vi "Configure Power.vi"(0 "VISA resource name":refnum<visa-resource-name>, 1 "Power Reference (0 dBm)":dbl, 2 "Enable Power Reference (F:Disable)":bool, 5 "Power (-130 dBm)":dbl=-130.0, 7 "Power Offset (0 dB)":dbl, 9 "Attenuator Auto Mode (T:Enable)":bool=TRUE, 11 "error in (no error)":errorcluster, 12 "Enable Attenuator Bypass (F:Disable)":bool, 13 "Attenuation Level (115 dB)":dbl=115.0) -> (4 "VISA resource name out":refnum<visa-resource-name>, 15 "error out":errorcluster)   [LabVIEW 2009, in "Agilent PSG MXG Series.lvlib"]
doc: "Configures RF output power."
uses:
  Agilent PSG MXG Series.lvlib
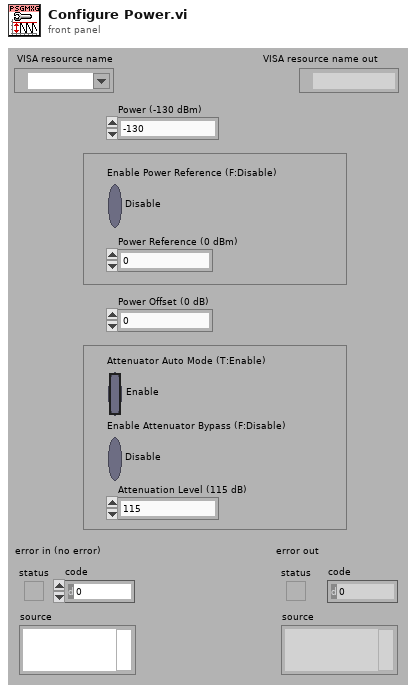
[diagram p1: front panel]
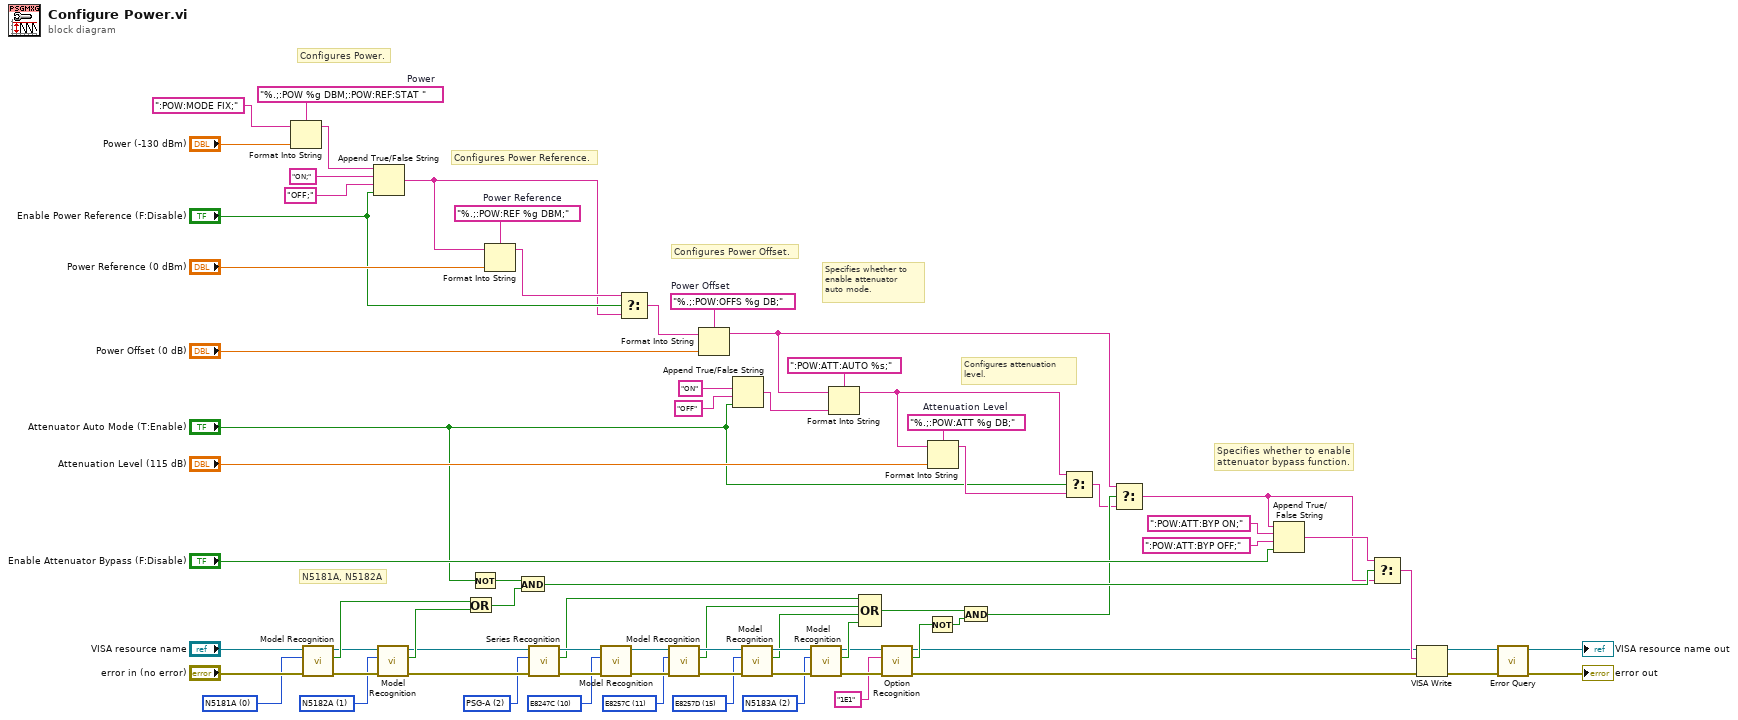
[diagram p0: block diagram]
diagram:
  w20 = u16 2 items=["N5181A"=0, "N5182A"=1, "N5183A"=2, "E8241A"=5, "E8244A"=6, "E8251A"=7, "E8254A"=8, "E8247C"=10, "E8257C"=11, "E8267C"=12, "E8257D"=15, "E8267D"=16] ("Model Type (0: N5181A)")
  w23 = u16 15 items=["N5181A"=0, "N5182A"=1, "N5183A"=2, "E8241A"=5, "E8244A"=6, "E8251A"=7, "E8254A"=8, "E8247C"=10, "E8257C"=11, "E8267C"=12, "E8257D"=15, "E8267D"=16] ("Model Type (0: N5181A)")
  w26 = u16 11 items=["N5181A"=0, "N5182A"=1, "N5183A"=2, "E8241A"=5, "E8244A"=6, "E8251A"=7, "E8254A"=8, "E8247C"=10, "E8257C"=11, "E8267C"=12, "E8257D"=15, "E8267D"=16] ("Model Type (0: N5181A)")
  w29 = u16 10 items=["N5181A"=0, "N5182A"=1, "N5183A"=2, "E8241A"=5, "E8244A"=6, "E8251A"=7, "E8254A"=8, "E8247C"=10, "E8257C"=11, "E8267C"=12, "E8257D"=15, "E8267D"=16] ("Model Type (0: N5181A)")
  w32 = u16 2 items=["MXG", "PSG", "PSG-A", "PSG-C", "PSG-D"] ("Series Type (0: MXG)")
  w36 = u16 1 items=["N5181A"=0, "N5182A"=1, "N5183A"=2, "E8241A"=5, "E8244A"=6, "E8251A"=7, "E8254A"=8, "E8247C"=10, "E8257C"=11, "E8267C"=12, "E8257D"=15, "E8267D"=16] ("Model Type (0: N5181A)")
  w41 = u16 0 items=["N5181A"=0, "N5182A"=1, "N5183A"=2, "E8241A"=5, "E8244A"=6, "E8251A"=7, "E8254A"=8, "E8247C"=10, "E8257C"=11, "E8267C"=12, "E8257D"=15, "E8267D"=16] ("Model Type (0: N5181A)")
  w51 = "%.;:POW:OFFS %g DB;"  # Power Offset
  w66 = "%.;:POW:ATT %g DB;"  # Attenuation Level
  w69 = "%.;:POW:REF %g DBM;"  # Power Reference
  w74 = "%.;:POW %g DBM;:POW:REF:STAT "  # Power
  # "N5181A, N5182A"
  # "Specifies whether to enable\nattenuator bypass function."
  # "Configures attenuation\nlevel."
  # "Specifies whether to\nenable attenuator\nauto mode."
  # "Configures Power Offset."
  # "Configures Power Reference."
  # "Configures Power."
  n1 = Format Into String(format string=w74, initial string=":POW:MODE FIX;" ("Power Mode"), "Power (-130 dBm)") -> (resulting string=w72:string)  [unwired: 1 in, 1 out]
  n2 = call "Model Recognition.vi"("error in (no error)"="error in (no error)", "Model Type (0: N5181A)"=w41, "VISA resource name"="VISA resource name") -> ("error out"=w37:errorcluster, "Is Model Correct"=w39:bool, "VISA resource name out"=w38:refnum<visa-resource-name>)  [unwired: 6 out]
  n3 = Append True/False String(1:"Enable Power Reference (F:Disable)", 2:"OFF;" ("false string"), 3:"ON;" ("true string"), 4:w72) -> (0:w54:string)
  n4 = call "Model Recognition.vi"("error in (no error)"=w37, "Model Type (0: N5181A)"=w36, "VISA resource name"=w38) -> ("error out"=w33:errorcluster, "Is Model Correct"=w35:bool, "VISA resource name out"=w34:refnum<visa-resource-name>)  [unwired: 6 out]
  n5 = Or(x=w39, y=w35) -> (x .or. y?=w40:bool)
  n6 = Not(x="Attenuator Auto Mode (T:Enable)") -> (.not. x?=w49:bool)
  n7 = Format Into String(format string=w69, initial string=w54, "Power Reference (0 dBm)") -> (resulting string=w55:string)  [unwired: 1 in, 1 out]
  n8 = And(x=w49, y=w40) -> (x .and. y?=w57:bool)
  n9 = call "Series Recognition.vi"("error in (no error)"=w33, "Series Type (0: MXG)"=w32, "VISA resource name"=w34) -> ("error out"=w30:errorcluster, "Is Series Correct"=w19:bool, "VISA resource name out"=w31:refnum<visa-resource-name>)  [unwired: 6 out]
  n10 = call "Model Recognition.vi"("error in (no error)"=w30, "Model Type (0: N5181A)"=w29, "VISA resource name"=w31) -> ("error out"=w27:errorcluster, "VISA resource name out"=w28:refnum<visa-resource-name>)  [unwired: 7 out]
  n11 = Select(t=w55, s="Enable Power Reference (F:Disable)", f=w54) -> (s? t:f=w52:string)
  n12 = call "Model Recognition.vi"("error in (no error)"=w27, "Model Type (0: N5181A)"=w26, "VISA resource name"=w28) -> ("error out"=w24:errorcluster, "Is Model Correct"=w18:bool, "VISA resource name out"=w25:refnum<visa-resource-name>)  [unwired: 6 out]
  n13 = Format Into String(format string=w51, initial string=w52, "Power Offset (0 dB)") -> (resulting string=w5:string)  [unwired: 1 in, 1 out]
  n14 = Append True/False String(1:"Attenuator Auto Mode (T:Enable)", 2:"OFF" ("false string"), 3:"ON" ("true string")) -> (0:w10:string)  [unwired: 1 out]
  n15 = call "Model Recognition.vi"("error in (no error)"=w24, "Model Type (0: N5181A)"=w23, "VISA resource name"=w25) -> ("error out"=w21:errorcluster, "Is Model Correct"=w17:bool, "VISA resource name out"=w22:refnum<visa-resource-name>)  [unwired: 6 out]
  n16 = call "Model Recognition.vi"("error in (no error)"=w21, "Model Type (0: N5181A)"=w20, "VISA resource name"=w22) -> ("error out"=w14:errorcluster, "Is Model Correct"=w16:bool, "VISA resource name out"=w15:refnum<visa-resource-name>)  [unwired: 6 out]
  n17 = Format Into String(format string=":POW:ATT:AUTO %s;", initial string=w5, w10) -> (resulting string=w9:string)  [unwired: 1 in, 1 out]
  n18 = Compound Arithmetic op=OR(w19, w18, w17, w16) -> (w12:bool)
  n19 = call "Option Recognition.vi"("error in (no error)"=w14, "Option (\"\")"="1E1" ("Option (\"\")"), "VISA resource name"=w15) -> ("error out"=w1:errorcluster, "Is Option Installed"=w6:bool, "VISA resource name out"=w2:refnum<visa-resource-name>)  [unwired: 6 out]
  n20 = Not(x=w6) -> (.not. x?=w7:bool)
  n21 = Format Into String(format string=w66, initial string=w9, "Attenuation Level (115 dB)") -> (resulting string=w64:string)  [unwired: 1 in, 1 out]
  n22 = And(x=w12, y=w7) -> (x .and. y?=w8:bool)
  n23 = Select(t=w9, s="Attenuator Auto Mode (T:Enable)", f=w64) -> (s? t:f=w4:string)
  n24 = Select(t=w5, s=w8, f=w4) -> (s? t:f=w3:string)
  n25 = Append True/False String(1:"Enable Attenuator Bypass (F:Disable)", 2:":POW:ATT:BYP OFF;" ("true string"), 3:":POW:ATT:BYP ON;" ("true string"), 4:w3) -> (0:w47:string)
  n26 = Select(t=w47, s=w57, f=w3) -> (s? t:f=w59:string)
  n27 = VISA Write(VISA resource name=w2, write buffer=w59, error in (no error)=w1) -> (VISA resource name out=w61:refnum<visa-resource-name>, error out=w60:errorcluster)  [unwired: 1 out]
  n28 = call "Error Query.vi"("error in (no error)"=w60, "VISA resource name"=w61) -> ("error out"=→"error out":errorcluster, "VISA resource name out"=→"VISA resource name out":refnum<visa-resource-name>)  [unwired: 8 out]
